vi "Actuate HW.vi"(8 "error in (no error)":errorcluster, 11 "Simulated Servo in":refnum<class "Simulated Servo.lvclass">) -> (0 "error out":errorcluster, 3 "Simulated Servo out":refnum<class "Simulated Servo.lvclass">)   [LabVIEW 2020, in "Simulated Servo.lvclass"]
uses:
  Simulated Servo.lvclass
  C:/Users/jharw/Documents/1 Folder to Rule them All/UMD/Inflation-Apparatus/src/Hardware/General Hardware.lvclass
  C:/Users/jharw/Documents/1 Folder to Rule them All/UMD/Inflation-Apparatus/src/Hardware/Actuators/Servos/Servo.lvclass
  General Hardware.lvclass/General Hardware.ctl
  Servo.lvclass/Servo.ctl
  <vilib>/numeric/Random Number (Range) DBL.vi
  Servo.lvclass
  General Hardware.lvclass
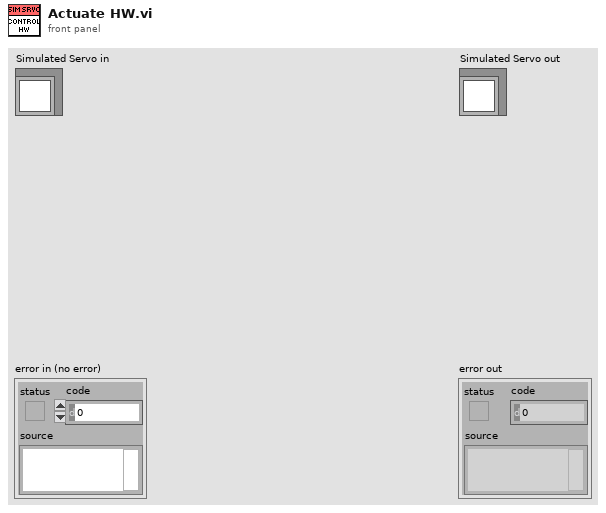
[diagram p1: front panel]
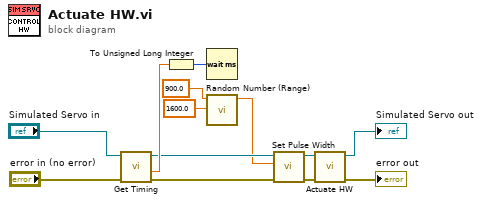
[diagram p0: block diagram]
diagram:
  n1 = call "Get Timing.vi"("error in (no error)"="error in (no error)", "General Hardware in"="Simulated Servo in") -> ("error out"=w8:errorcluster, "time delay (ms)"=w10:dbl, "General Hardware out"=w9:refnum<class "Simulated Servo.lvclass">)  [unwired: 6 in, 1 out]
  n2 = To Unsigned Long Integer(number=w10) -> (unsigned 32bit integer=w11:u32)
  n3 = Wait (ms)(milliseconds to wait=w11) -> ()  [unwired: 1 out]
  n4 = call-poly <vilib>:"Random Number (Range).vi"("lower bound (0)"=1600.0, "upper bound (100)"=900.0) -> ("number"=w2:dbl)  [unwired: 9 in]
  n5 = call "Set Pulse Width.vi"("error in (no error)"=w8, "pulse width (micro-sec)"=w2, "Servo in"=w9) -> ("error out"=w7:errorcluster, "Servo out"=w5:refnum<class "Simulated Servo.lvclass">)  [unwired: 7 in]
  n6 = call-parent "Actuate HW.vi"("error in (no error)"=w7, "Servo in"=w5) -> ("error out"=→"error out":errorcluster, "Servo out"=→"Simulated Servo out":refnum<class "Simulated Servo.lvclass">)  [unwired: 8 in]
